vi "SubVI_SaveAsTXT.vi"(6 "Range Slide":cluster{dbl, dbl}={0.0, 1.0}, 8 "error in":errorcluster, 9 "Channel Selection":bool[](array[boolean]), 11 "source file path":path=path "D:/Desktop/A  2013-0104-1030-14.txt") -> (0 "error out":errorcluster)   [LabVIEW 2011]
uses:
  <vilib>/Utility/file.llb/Write To Spreadsheet File (string).vi
panel:
  out "Numeric":i32
  out "target file path":path=path "D:/Desktop/A  2013-0104-1030-14.A.txt"
  out "End(1.0)":dbl=1.0
  out "Start(0.0)":dbl
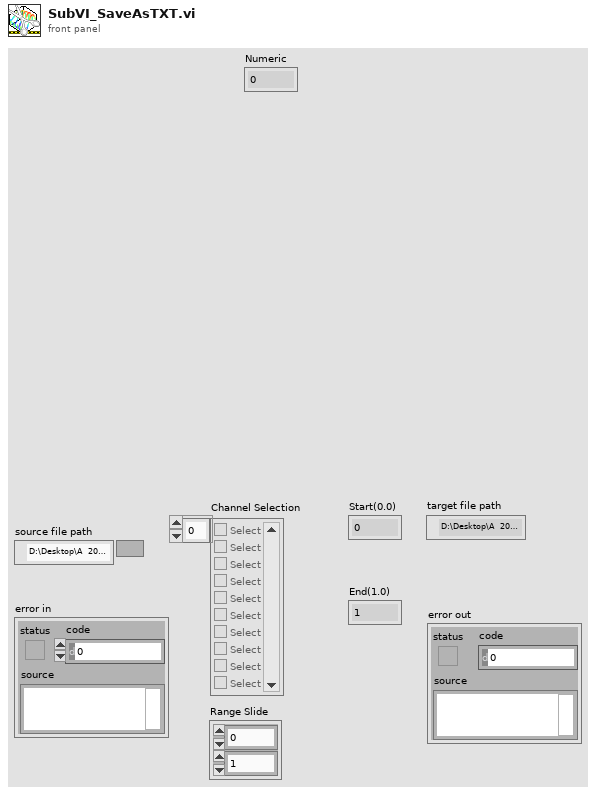
[diagram p1: front panel]
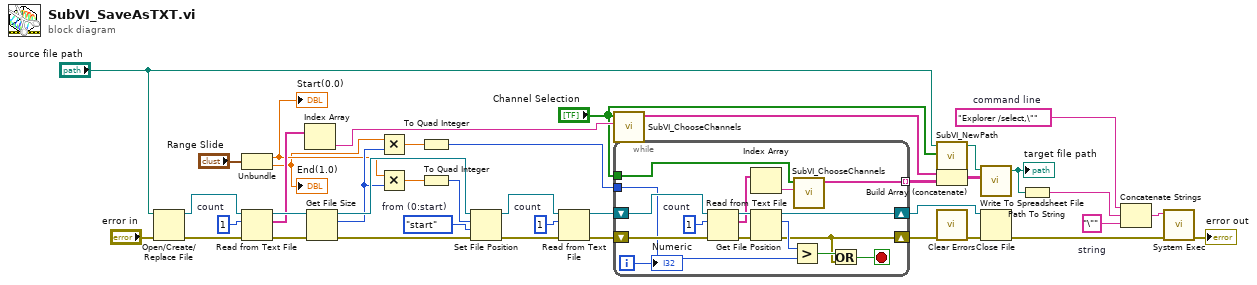
[diagram p0: block diagram]
diagram:
  w7 = "\""  # string
  w10 = "Explorer /select,\""  # command line
  w24 = 1  # count
  w37 = 1  # count
  w38 = enum16{"start", "end", "current"}."start"  # from (0:start)
  n1 = Open/Create/Replace File(file path (use dialog)="source file path", error in="error in") -> (refnum out=w36:refnum<file>, error out=w34:errorcluster)  [unwired: 4 in, 1 out]
  n2 = Unbundle("Range Slide") -> (w14:dbl, w13:dbl)
  "Start(0.0)" <- w14
  "End(1.0)" <- w13
  n3 = Read from Text File(file (use dialog)=w36, count=w37, error in=w34) -> (refnum out=w35:refnum<file>, text=w18:string[], error out=w33:errorcluster)  [unwired: 1 in, 1 out]
  n4 = Index Array(array=w18) -> (element=w19:string)  [unwired: 1 in]
  n5 = Get File Size(file=w35, error in=w33) -> (refnum out=w32:refnum<file>, size (in bytes)=w27:i64, 0:w31:errorcluster)
  n6 = Multiply(x=w13, y=w27) -> (x*y=w28:dbl)
  n7 = Multiply(x=w14, y=w27) -> (x*y=w30:dbl)
  n8 = To Quad Integer(1:w28) -> (0:w26:i64)
  n9 = To Quad Integer(1:w30) -> (0:w29:i64)
  n10 = Set File Position(offset (in bytes) (0)=w29, refnum=w32, from (0:start)=w38, error in=w31) -> (refnum out=w23:refnum<file>, error out=w21:errorcluster)
  n11 = Read from Text File(file (use dialog)=w23, count=w24, error in=w21) -> (refnum out=w22:refnum<file>, error out=w20:errorcluster)  [unwired: 1 in, 2 out]
  n12 = call "SubVI_ChooseChannels.vi"("String"=w19, "Channel Selection"="Channel Selection") -> ("Array"=w16:string[])  [unwired: 9 in]
  n13 = while {
    shift-right: [w50] -> w40
    shift-left: w22 -> [w52]
    shift-right: [w42] -> w39
    shift-left: w20 -> [w51]
    tunnel: w26 -> [w47]
    tunnel: [w45] -> w25 mode=indexing
    tunnel: "Channel Selection" -> [w44]
    i -> [w41]
    stop <- w43 stop-if-true
    w56 = 1  # count
    n14 = Read from Text File(file (use dialog)=w52, count=w56, error in=w51) -> (refnum out=w55:refnum<file>, text=w54:string[], error out=w49:errorcluster)  [unwired: 1 in, 1 out]
    n15 = Index Array(array=w54) -> (element=w53:string)  [unwired: 1 in]
    n16 = Get File Position(4:w49, 7:w55) -> (0:w42:errorcluster, 2:w48:i64, 3:w50:refnum<file>)
    n17 = Greater?(x=w48, y=w47) -> (0:w46:bool)
    n18 = call "SubVI_ChooseChannels.vi"("String"=w53, "Channel Selection"=w44) -> ("Array"=w45:string[])  [unwired: 9 in]
    n19 = Or(x=w46, y=w42) -> (x .or. y?=w43:bool)
    "Numeric" <- w41
  }
  n20 = call "SubVI_NewPath.vi"("Channel Selection"="Channel Selection", "source file path"="source file path") -> ("New file path"=w6:path)  [unwired: 9 in]
  n21 = Build Array (concatenate)(w16, w25) -> (w17:string[][])
  n22 = call <vilib>:"Clear Errors.vi"("error in (no error)"=w39) -> ("error out"=w1:errorcluster)  [unwired: 6 in]
  n23 = call-poly <vilib>:"Write To Spreadsheet File.vi"("2D data"=w17, "file path (dialog if empty)"=w6) -> ("new file path (Not A Path if cancelled)"=w5:path)  [unwired: 6 in]
  "target file path" <- w5
  n24 = Close File(refnum=w40, error in=w1) -> (error out=w4:errorcluster)  [unwired: 1 out]
  n25 = Path To String(path=w5) -> (string=w8:string)
  n26 = Concatenate Strings(w10, w8, w7) -> (w9:string)
  n27 = call <vilib>:"System Exec.vi"("error in (no error)"=w4, "command line"=w9) -> ("error out"=→"error out":errorcluster)  [unwired: 6 in, 3 out]
